vi "T564_TriggerLevelFromSETresponse.vi"(11 "StringIn":string) -> (3 "TriggerLevel":string)   [LabVIEW 2020]
uses:
  Match Regular Expression.xnode
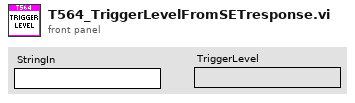
[diagram p1: front panel]
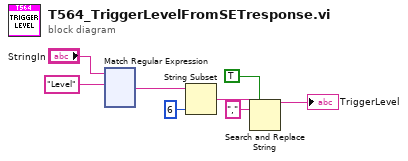
[diagram p0: block diagram]
diagram:
  n1 = xnode "Match Regular Expression"("input string"="StringIn", "regular expression"="Level") -> ("after match"=w4:string)  [unwired: 4 in, 4 out]
  n2 = String Subset(string=w4, length (rest)=6 ("length (rest)")) -> (substring=w6:string)  [unwired: 1 in]
  n3 = Search and Replace String(replace all?=TRUE ("replace all? (F)"), input string=w6, search string=",") -> (result string=→"TriggerLevel":string)  [unwired: 5 in, 3 out]
